vi "pointbypointvi.vi"() -> ()   [LabVIEW 2016]
uses:
  <vilib>/ptbypt/NI_PtbyPt.lvlib
panel:
  out "appended array":dbl[][](array[numeric])
  out "Waveform Graph":dbl[](graph)
  out "Waveform Chart":dbl(graph)
  in  "stop":bool
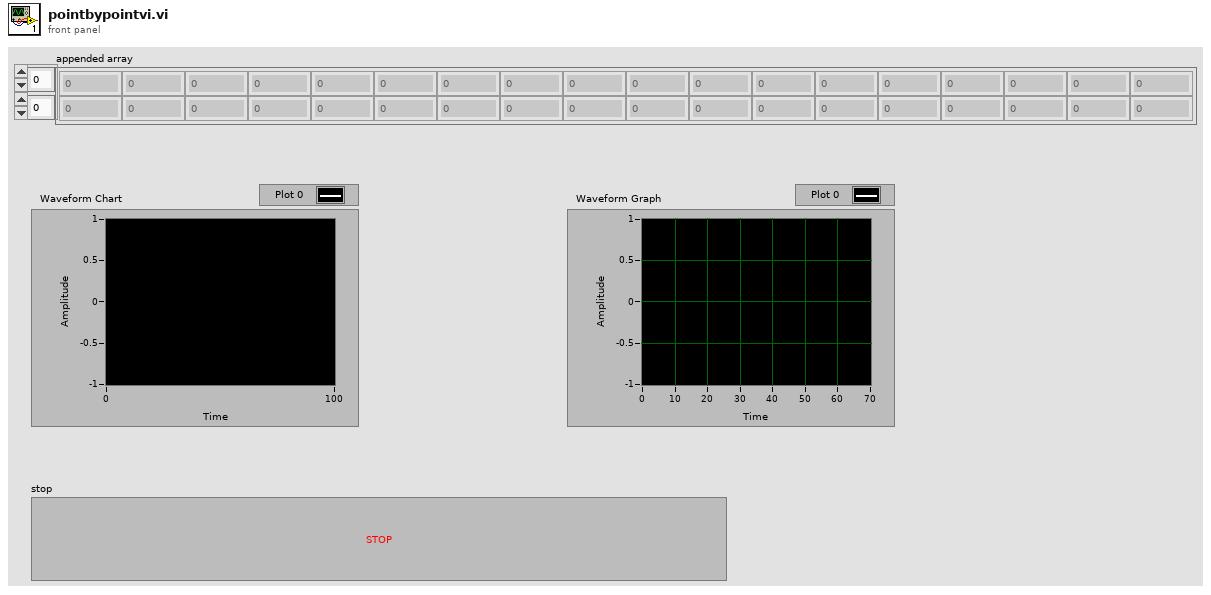
[diagram p1: front panel]
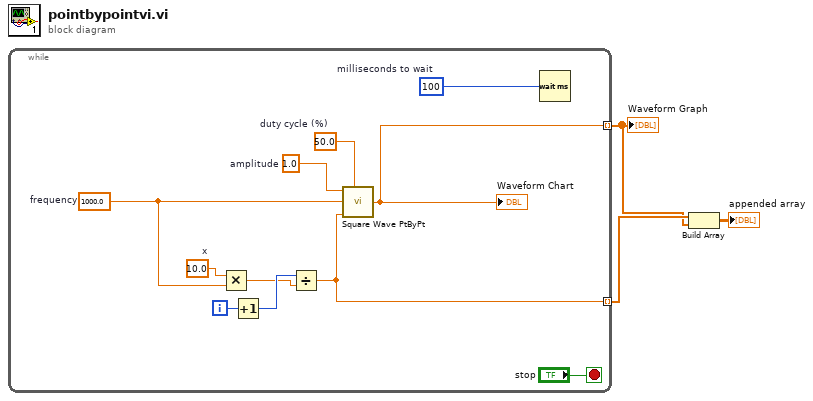
[diagram p0: block diagram]
diagram:
  n1 = while {
    tunnel: [w9] -> w2 mode=indexing
    tunnel: [w7] -> w3 mode=indexing
    i -> [w11]
    stop <- "stop" stop-if-true
    w4 = 10.0  # x
    w10 = u32 100  # milliseconds to wait
    w6 = 1000.0  # frequency
    w12 = 1.0  # amplitude
    w13 = 50.0  # duty cycle (%)
    n2 = Multiply(x=w4, y=w6) -> (x*y=w5:dbl)
    n3 = Increment(x=w11) -> (x+1=w8:i32)
    n4 = Divide(x=w8, y=w5) -> (x/y=w7:dbl)
    n5 = call <vilib>:"Square Wave PtByPt.vi"("amplitude"=w12, "frequency"=w6, "time"=w7, "duty cycle (%)"=w13) -> ("square wave"=w9:dbl)  [unwired: 1 in]
    "Waveform Chart" <- w9
    n6 = Wait (ms)(milliseconds to wait=w10) -> ()  [unwired: 1 out]
  }
  "Waveform Graph" <- w2
  n7 = Build Array(w3, w2) -> (→"appended array":dbl[][])
